vi "Set_FreqHist_Range.vi"(7 "Slide":cluster{dbl, dbl}, 9 "View Subset":bool, 11 "Freq HistoryRef":refnum<vi>) -> ()   [LabVIEW 2018]
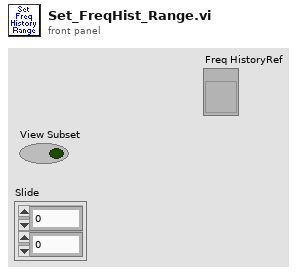
[diagram p1: front panel]
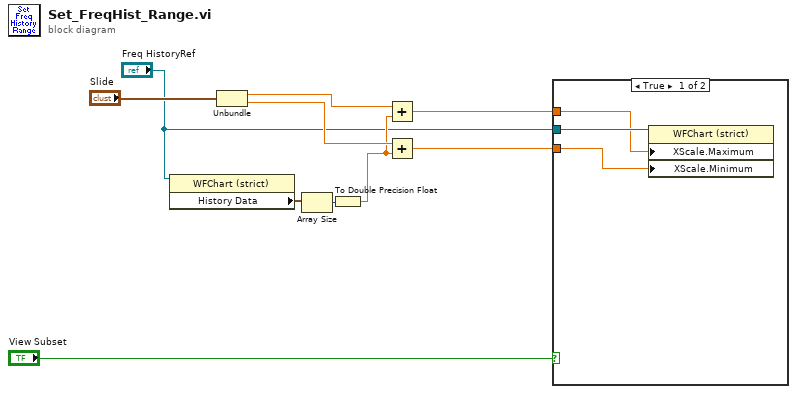
[diagram p0: block diagram]
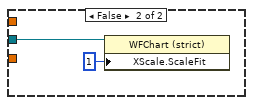
[diagram p2: hidden frame]
diagram:
  n1 = property class="WFChart (strict)"(reference="Freq HistoryRef") -> ("History Data"=w3:cluster{dbl, dbl, dbl}[])  [unwired: 1 in, 2 out]
  n2 = Unbundle("Slide") -> (w8:dbl, w10:dbl)
  n3 = Array Size(array=w3) -> (size(s)=w4:i32)
  n4 = To Double Precision Float(number=w4) -> (double precision float=w7:dbl)
  n5 = Add(x=w8, y=w7) -> (x+y=w5:dbl)
  n6 = Add(x=w10, y=w7) -> (x+y=w6:dbl)
  n7 = case shown="True" "View Subset" {
    tunnel: "Freq HistoryRef" -> [w13 w15]
    tunnel: w5 -> [w12 _]
    tunnel: w6 -> [w11 _]
    frame True {
      n8 = property class="WFChart (strict)"(reference=w13, "XScale.Maximum"=w12, "XScale.Minimum"=w11) -> ()  [unwired: 1 in, 2 out]
    }
    frame False {
      n9 = property class="WFChart (strict)"(reference=w15, "XScale.ScaleFit"=u8 1 ("X Scale.Scale Fit")) -> ()  [unwired: 1 in, 2 out]
    }
  }
